vi "MyRIO_Main.vi"   [LabVIEW 2019]
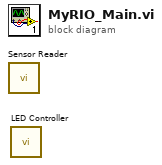
[diagram p0: block diagram]
diagram:
  n1 = call "Sensor Reader.vi"() -> ()  [unwired: 12 in]
  n2 = call "LED Controller.vi"() -> ()  [unwired: 12 in]
